vi "raptor_stop.vi"(8 "error in (no error)":errorcluster) -> (0 "error out":errorcluster)   [LabVIEW 2016]
doc: "Raptor: Stops processing without ending scan."
uses:
  typedef/raptor_message.ctl
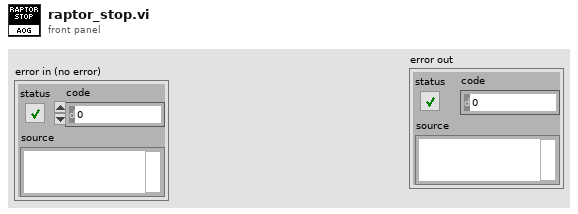
[diagram p1: front panel]
types:
  T1 = typedef "raptor_message.ctl" = cluster{"Message":enum16{"start", "stop", "initialise", "shutdown", "end scan", "new scan", "set depth"}, "Data":variant}
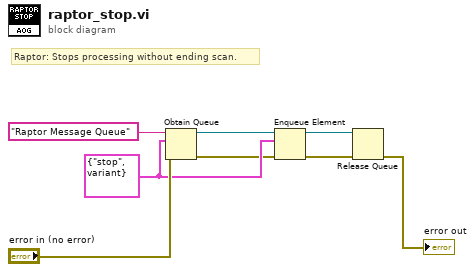
[diagram p0: block diagram]
diagram:
  w5 = T1 {"Message"=enum."stop", "Data"=variant} ("Cluster")
  # "Raptor: Stops processing without ending scan."
  n1 = Obtain Queue(name (unnamed)="Raptor Message Queue", element data type=w5, error in (no error)="error in (no error)") -> (queue out=w6:refnum<queue>, error out=w2:errorcluster)  [unwired: 2 in, 1 out]
  n2 = Enqueue Element(queue=w6, element=w5, error in (no error)=w2) -> (queue out=w4:refnum<queue>, error out=w3:errorcluster)  [unwired: 1 in, 1 out]
  n3 = Release Queue(queue=w4, error in (no error)=w3) -> (error out=→"error out":errorcluster)  [unwired: 1 in, 2 out]
